vi "Material-ConfigPage-SendMessageToContainer.vi"(0 "Configuration Page":refnum<class "Material-ConfigPage.lvclass">, 5 "Parameter":string, 7 "Payload":variant, 11 "error in":errorcluster) -> (4 "Configuration Page out":refnum<class "Material-ConfigPage.lvclass">, 15 "error out":errorcluster)   [LabVIEW 2013, in "Material-ConfigPage.lvclass"]
uses:
  Material-ConfigPage.lvclass
  Material-ConfigPage.lvclass/Material-ConfigPage.ctl
  Reuse Library/featherweight/Core/Messaging/Messenger.Actor/FTW-Messenger-Actor.lvclass
panel:
  # "Inputs"
  # "Outputs"
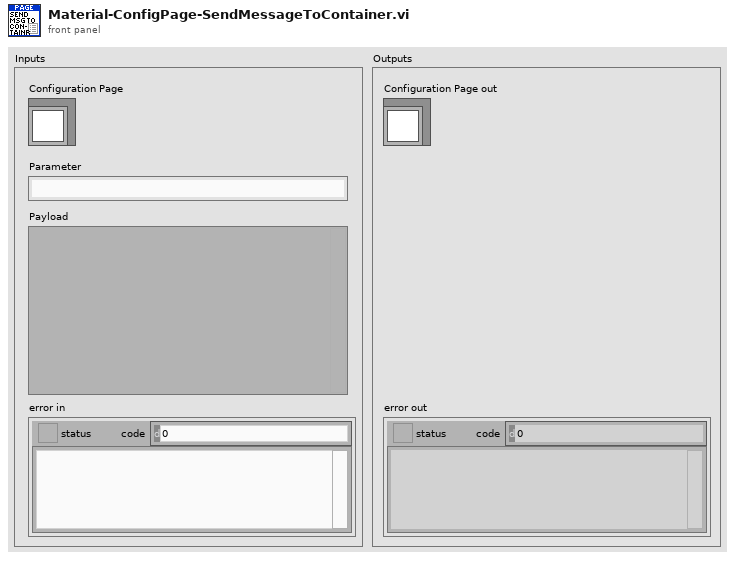
[diagram p1: front panel]
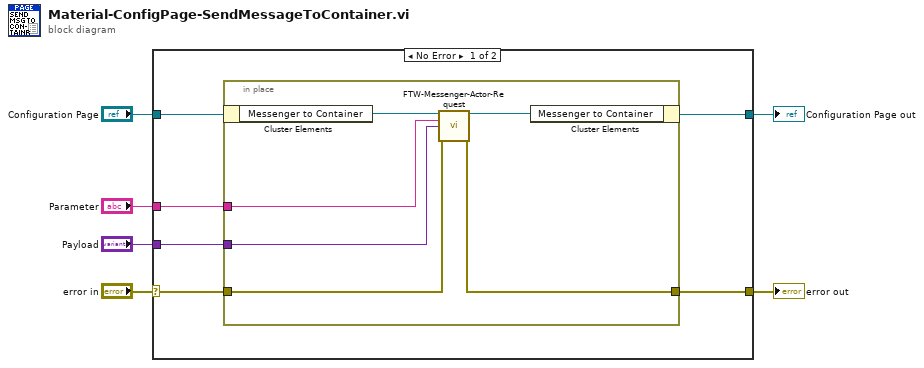
[diagram p0: block diagram]
diagram:
  n1 = case shown="No Error" "error in" {
    selector: "error in" -> [w10 w20]
    tunnel: [w9 w20] -> w6
    tunnel: [w7 w19] -> w4
    tunnel: "Configuration Page" -> [w8 w19]
    tunnel: "Parameter" -> [w12 _]
    tunnel: "Payload" -> [w11 _]
    frame No Error {
      n2 = in-place {
        in-place-border: w12 -> [w18]
        in-place-border: w11 -> [w17]
        in-place-border: w10 -> [w16]
        in-place-border: [w15] -> w9
        n3 = in-place-cluster #1(w8) -> ("Messenger to Container"=w14:refnum<class "FTW-Messenger-Actor.lvclass">)
        n4 = call-dynamic "FTW-Messenger-Actor-Request.vi"("Messenger"=w14, "Parameter"=w18, "Payload"=w17, "error in"=w16) -> ("Messenger out"=w13:refnum<class "FTW-Messenger-Actor.lvclass">, "error out"=w15:errorcluster)  [unwired: 10 in]
        n5 = in-place-cluster #1("Messenger to Container"=w13) -> (w7:refnum<class "Material-ConfigPage.lvclass">)
      }
    }
    frame Error {
    }
  }
  "error out" <- w6
  "Configuration Page out" <- w4
